vi "MoveToPosition2.vi"(7 "In Contact in":bool, 10 "Position in":bool, 11 "UiDefinition 2":T1) -> (3 "In Contact out":bool)   [LabVIEW 2020]
uses:
  UIReferences.ctl
  C:/Projects/RaxTagServer/LabviewDXFViewer/LabviewDXFViewer/bin/Release/LabviewDXFViewer.exe
  LabviewDXFViewer/bin/Release/LabviewDXFViewer.exe
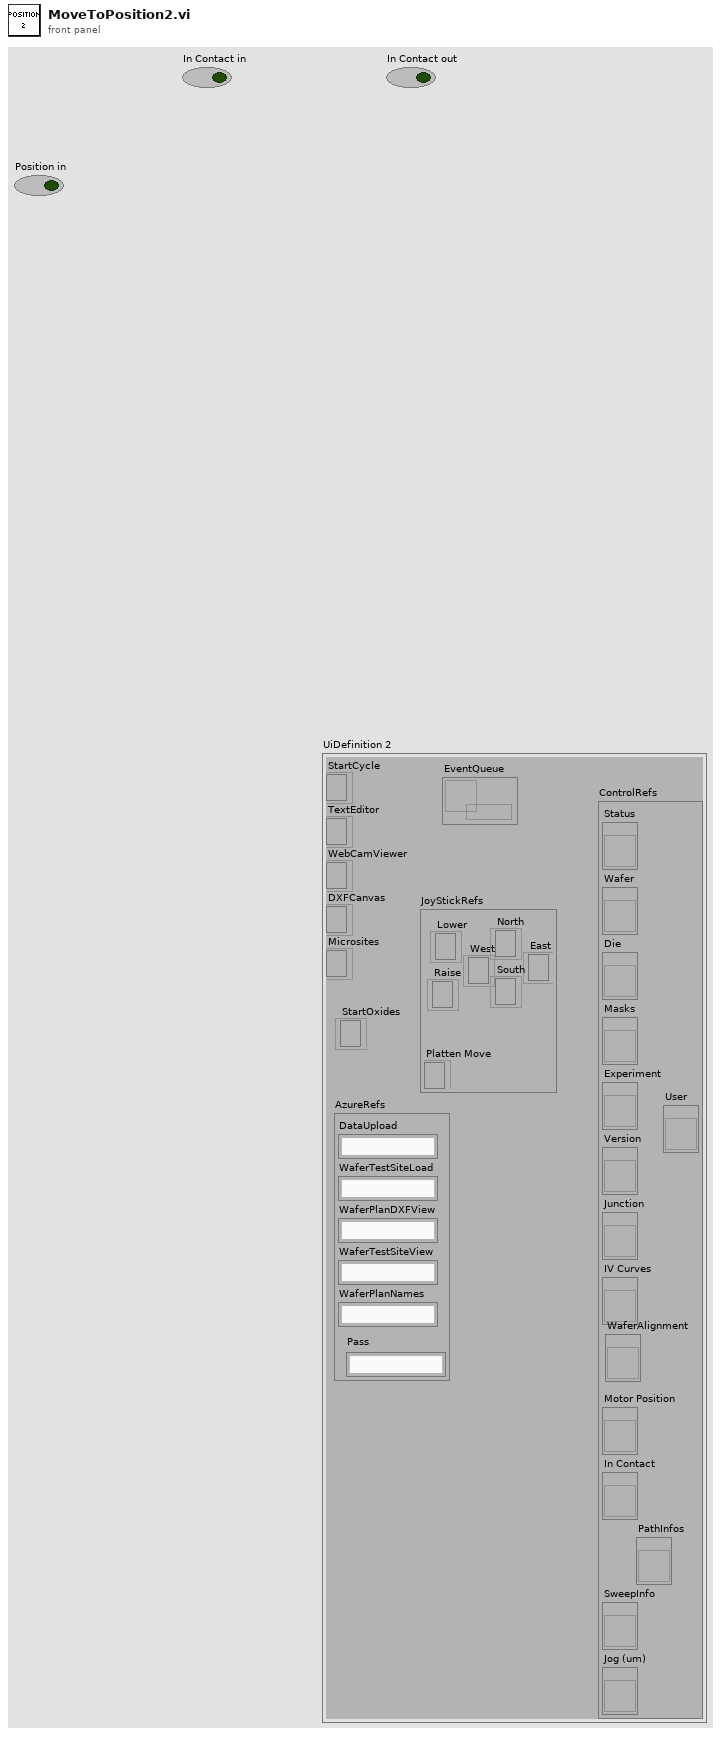
[diagram p1: front panel]
types:
  T1 = typedef "UIReferences.ctl" = cluster{"StartCycle":refnum<k24>, "TextEditor":refnum<k24>, "WebCamViewer":refnum<k24>, "DXFCanvas":refnum<k24>, "Microsites":refnum<k24>, "JoyStickRefs":cluster{"North":refnum<k24>, "Lower":refnum<k24>, "Raise":refnum<k24>, "Platten Move":refnum<k24>, "West":refnum<k24>, "East":refnum<k24>, "South":refnum<k24>}, "AzureRefs":cluster{"DataUpload":string, "WaferTestSiteLoad":string, "WaferPlanDXFView":string, "WaferTestSiteView":string, "WaferPlanNames":string, "Pass":string}, "ControlRefs":cluster{"Status":refnum<vi>, "Wafer":refnum<vi>, "Die":refnum<vi>, "Masks":refnum<vi>, "Experiment":refnum<vi>, "Version":refnum<vi>, "Junction":refnum<vi>, "IV Curves":refnum<vi>, "Motor Position":refnum<vi>, "In Contact":refnum<vi>, "SweepInfo":refnum<vi>, "Jog (um)":refnum<vi>, "PathInfos":refnum<vi>, "User":refnum<vi>, "WaferAlignment":refnum<vi>}, "EventQueue":refnum<queue>, "StartOxides":refnum<k24>}
  T2 = typedef "WaferAlignmentType.ctl" = cluster{"Wafer Units to microns":dbl, "Rotation Misalign":dbl[], "Scale Misalign":dbl, "Steps Per micron":dbl, "Position 1":i32[], "Chip Orientation":i32, "Position 2":i32[], "Lift Distance":i32, "Position 3":i32[], "Jog Height":i32}
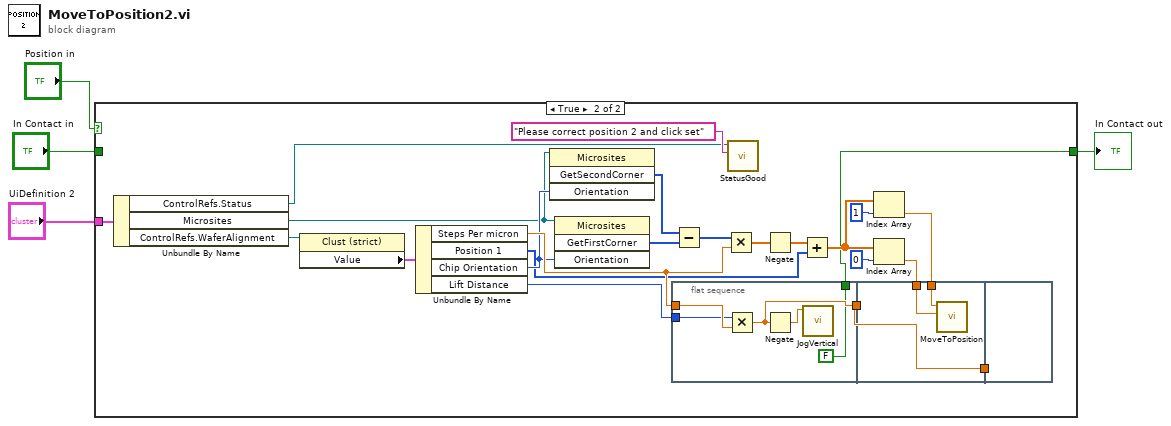
[diagram p0: block diagram]
diagram:
  n1 = case shown="True" "Position in" {
    tunnel: [w5 w11] -> w3
    tunnel: "In Contact in" -> [w5 _]
    tunnel: "UiDefinition 2" -> [_ w9]
    frame False {
    }
    frame True {
      n2 = Unbundle By Name(w9) -> ("ControlRefs.Status"=w7:refnum<vi>, "Microsites"=w6:refnum<k24>, "ControlRefs.WaferAlignment"=w10:refnum<vi>)
      n3 = property class="Clust (strict)"(reference=w10) -> ("Value"=w8:T2)  [unwired: 1 in, 2 out]
      n4 = Unbundle By Name(w8) -> ("Steps Per micron"=w15:dbl, "Position 1"=w13:i32[], "Chip Orientation"=w14:i32, "Lift Distance"=w12:i32)
      n5 = invoke class="Microsites" method="GetSecondCorner"(reference=w6, "Orientation"=w14) -> ("GetSecondCorner"=w28:i32[])  [unwired: 2 in, 3 out]
      n6 = invoke class="Microsites" method="GetFirstCorner"(reference=w6, "Orientation"=w14) -> ("GetFirstCorner"=w26:i32[])  [unwired: 2 in, 3 out]
      n7 = flat-sequence {
        tunnel: w15 -> [w32]
        tunnel: [w31] -> w21
        tunnel: w12 -> [w30]
        tunnel: [FALSE ("In Contact")] -> w11
        tunnel: w24 -> [w36]
        tunnel: w23 -> [w35]
        tunnel: [w34] -> w22
        tunnel: w21 -> [w34]
        tunnel: w22 -> [_]
        frame #0 {
          n8 = Multiply(x=w30, y=w32) -> (x*y=w31:dbl)
          n9 = Negate(x=w31) -> (-x=w33:dbl)
          n10 = call "JogVertical.vi"("Numeric"=w33) -> ()  [unwired: 11 in]
        }
        frame #1 {
          n11 = call "MoveToPosition.vi"("Y"=w36, "X"=w35) -> ()  [unwired: 10 in]
        }
        frame #2 {
        }
      }
      n12 = Subtract(x=w28, y=w26) -> (x-y=w27:i32[])
      n13 = Multiply(x=w27, y=w15) -> (x*y=w25:dbl[])
      n14 = call "StatusGood.vi"("Text.Text"="Please correct position 2 and click set" ("Status"), "String in"=w7) -> ()  [unwired: 10 in]
      n15 = Negate(x=w25) -> (-x=w17:dbl[])
      n16 = Add(x=w17, y=w13) -> (x+y=w18:dbl[])
      n17 = Index Array(array=w18, index=1) -> (element=w23:dbl)
      n18 = Index Array(array=w18, index=0) -> (element=w24:dbl)
    }
  }
  "In Contact out" <- w3
